vi "1,3A PWM-MotorControl and VBattSense FPGA.vi"() -> ()   [LabVIEW 2011]
doc: "FPGA VI for motor control and VBAttery Sensing.\n\nMotor Control:\nBoth servos are linked to seperate I/O terminals. The Generate Digital Pulse VI inouts the PUlsewidth in us (outputted by the 1.3A PWM Motor Control VI) and creates corresponding pulses on the pins. The clock timer determines the PWM cycle time."
uses:
  TestCode/spiTest/FPGA/Controls/Port Action.ctl
  <vilib>/Platform/TimedLoop/XDataNode/timing_clust.ctl
  <vilib>/Platform/TimedLoop/XDataNode/nitl_modes.ctl
  <vilib>/Platform/TimedLoop/XDataNode/wakeup.ctl
  <vilib>/robotics/Utilities/FPGA Utilities/Generate Digital Pulse (uSec).vi
  <vilib>/rvi/eio/common/nirviEmuTemplateMethod_errors.vi
  <vilib>/Platform/TimedLoop/XDataNode/XDataNode.xnode
  <vilib>/eio/EIONode/EIONode.xnode
  <vilib>/robotics/Utilities/FPGA Utilities/NI_Robotics_FPGA Utilities.lvlib
  <vilib>/Platform/TimedLoop/XDataNode/XDNodeRunTimeDep.lvlib
panel:
  out "VBatt Sense Iterations":i32
  out "Averaged bitstring":bool[](array[boolean])
  in  "VBatt samples to average":u16=30
  out "vBatt ADC bits":u16
  in  "stop VBatt Sense":bool
  in  "SERVO 2 Duty (uSec)":u32
  in  "stop PWM":bool
  in  "SERVO 1 Duty (uSec)":u32
  # "IF YOU HAVE TROUBLE RUNNING THIS: \ncheck if you're running it on FPGA target"
  # "Winch"
  # "Rudder"
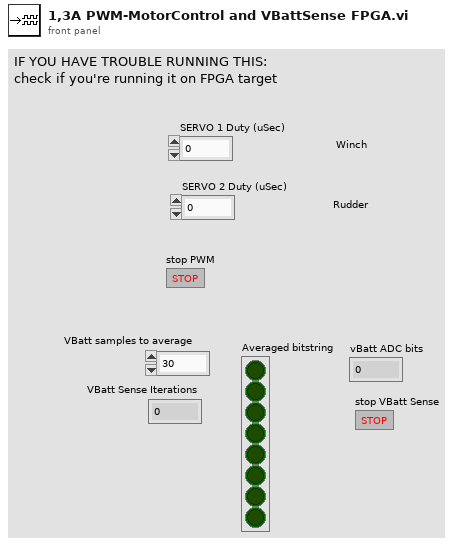
[diagram p1: front panel]
types:
  T1 = typedef "Port Action.ctl" = enum8{"Start Read", "Transition", "Wait Cycles", "End Read"}
  T2 = typedef "XDNodeRunTimeDep.lvlib/timing_clust.ctl" = cluster{"Expected End [f-1]":u64, "Actual End [f-1]":u64, "Finished Late? [f-1]":bool, "Expected End [i-1]":u64, "Actual End [i-1]":u64, "Finished Late? [i-1]":bool, "Expected Start [i]":u64, "Actual Start [i]":u64, "Expected Start [f]":u64, "Actual Start [f]":u64, "Source Name":string, "Structure Name":string, "Period":i64, "Deadline":i64, "Offset":i64, "Start":i64, "Priority":i32, "Timeout":i32, "Mode":T3, "Wakeup Reason":T4, "Error":errorcluster, "Source Type":string, "Secondary Source Type":string, "Global End Time":u64, "Global Start Time":u64, "Frame Duration":u64, "Iteration Duration":u64, "Assigned CPU":i32, "I/O Scan Engine Mode":u32}
  T3 = typedef "XDNodeRunTimeDep.lvlib/nitl_modes.ctl" = enum32{"No Change", "Process missed periods, maintain original phase", "Discard missed periods, maintain original phase", "Process missed periods, ignore original phase", "Discard missed periods, ignore original phase"}
  T4 = typedef "XDNodeRunTimeDep.lvlib/wakeup.ctl" = enum32{"Normal", "Aborted", "Asynchronous wakeup", "Timing source error", "Timed loop error", "Timeout"}
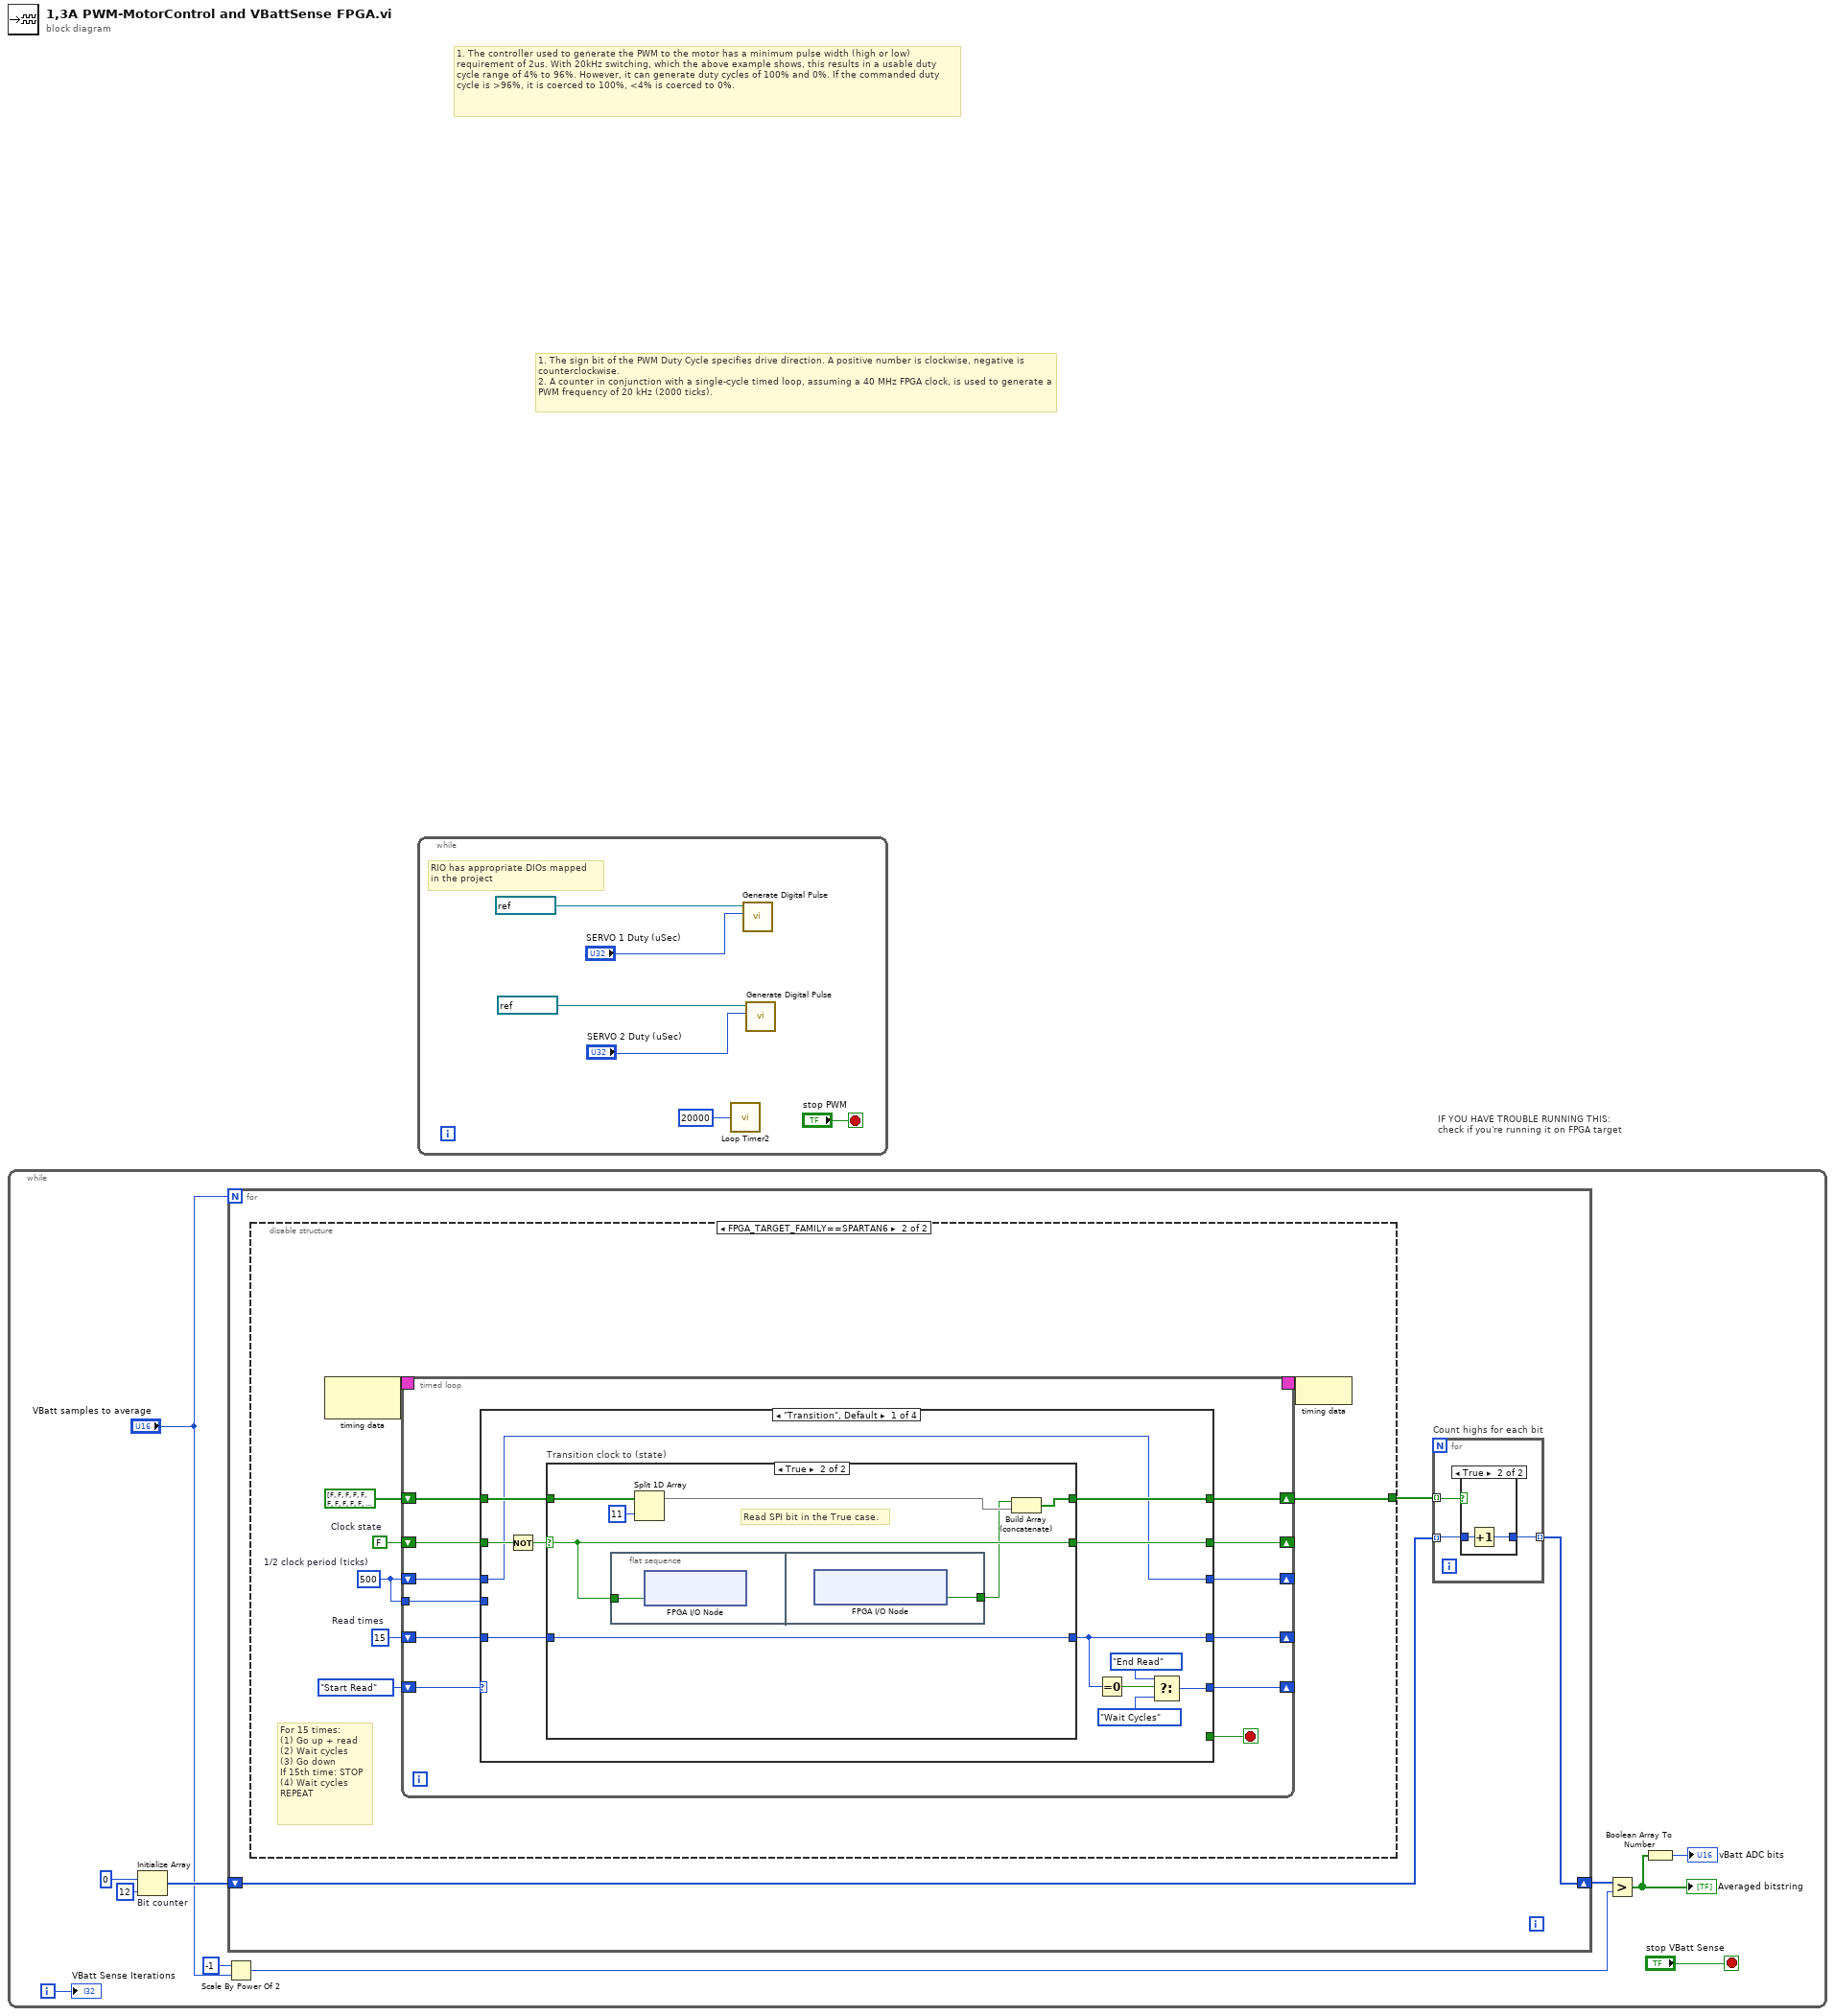
[diagram p0: block diagram]
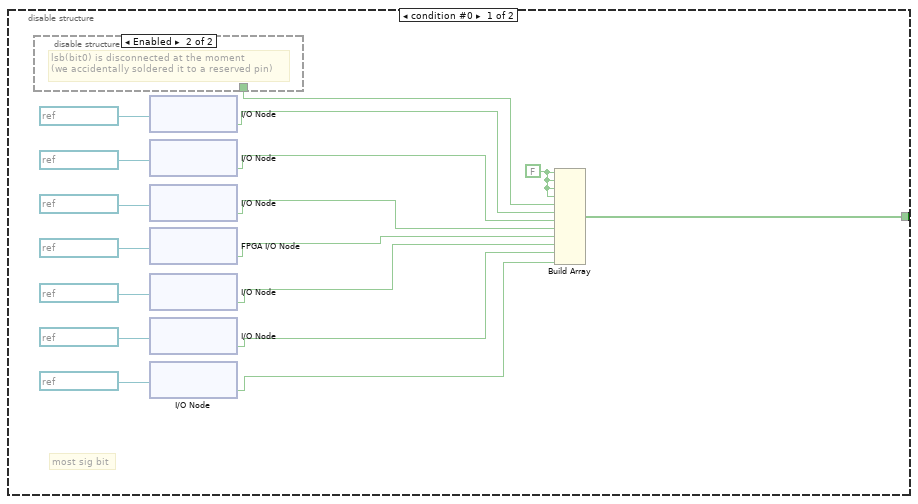
[diagram p2: hidden frame]
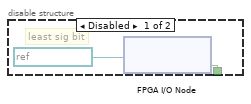
[diagram p3: hidden frame]
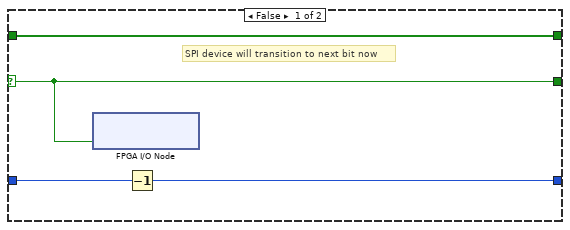
[diagram p4: hidden frame]
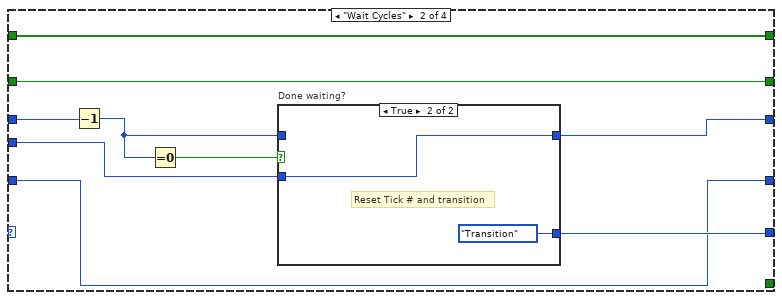
[diagram p5: hidden frame]
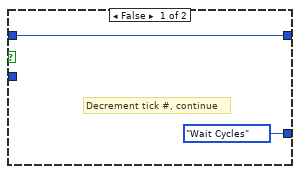
[diagram p6: hidden frame]
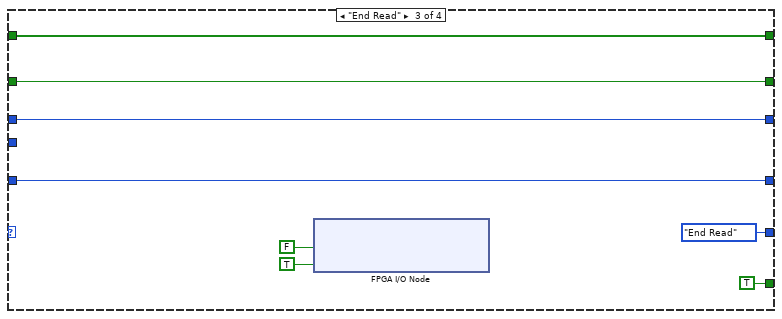
[diagram p7: hidden frame]
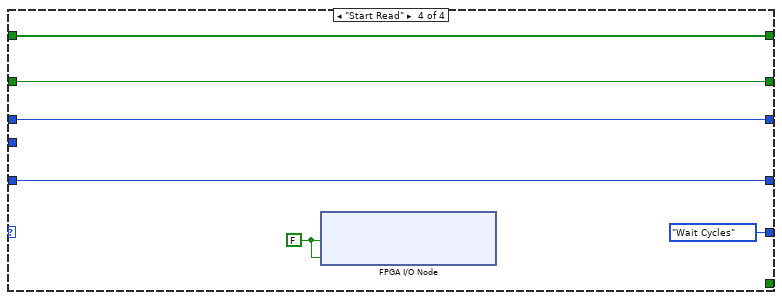
[diagram p8: hidden frame]
diagram:
  # "IF YOU HAVE TROUBLE RUNNING THIS: \ncheck if you're running it on FPGA target"
  # "1. The sign bit of the PWM Duty Cycle specifies drive direction. A positive number is clockwise, negative is counterclockwise.\n2. A counter in conjunction with a single-cycle timed loop, assuming a 40 MHz FPGA clock, is used to generate a PWM frequency of 20 kHz (2000 ticks)."
  # "1. The controller used to generate the PWM to the motor has a minimum pulse width (high or low) requirement of 2us. With 20kHz switching, which the above example shows, this results in a usable duty cycle range of 4% to 96%. However, it can generate duty cycles of 100% and 0%. If the commanded duty cycle is >96%, it is coerced to 100%, <4% is coerced to 0%."
  n1 = while {
    i -> [w8]
    stop <- "stop VBatt Sense" stop-if-true
    n2 = Initialize Array "Bit counter"(u16 0 ("VBatt Samples to read/2 2"), 12 ("dimension size")) -> (w5:u16[])
    n3 = Scale By Power Of 2(n=-1, x="VBatt samples to average") -> (x*2^n=w4:u16)
    n4 = for {
      N: "VBatt samples to average" -> [_]
      shift-right: [w12] -> w11
      shift-left: w5 -> [w14]
      n5 = disable-structure shown="FPGA_TARGET_FAMILY==SPARTAN6" {
        disable-tunnel: [w16 w34] -> w13
        frame condition #0 {
          w15 = FALSE ("element")
          # "most sig bit"
          n6 = disable-structure shown="Enabled" {
            disable-tunnel: [w32 _] -> w17
            frame Disabled {
              # "least sig bit"
              n7 = xnode "FPGA I/O Node"("FPGA I/O In"=refnum<k21> "VBatt bit0") -> ("I/O Item"=w32:bool)  [unwired: 1 out]
            }
            frame Enabled {
              # "lsb(bit0) is disconnected at the moment\n(we accidentally soldered it to a reserved pin)"
            }
          }
          n8 = xnode "I/O Node"("FPGA I/O In"=refnum<k21> "VBatt bit1") -> ("I/O Item"=w25:bool)  [unwired: 1 out]
          n9 = xnode "I/O Node"("FPGA I/O In"=refnum<k21> "VBatt bit2") -> ("I/O Item"=w26:bool)  [unwired: 1 out]
          n10 = xnode "I/O Node"("FPGA I/O In"=refnum<k21> "VBatt bit3") -> ("I/O Item"=w27:bool)  [unwired: 1 out]
          n11 = xnode "FPGA I/O Node"("FPGA I/O In"=refnum<k21> "VBatt bit4") -> ("I/O Item"=w28:bool)  [unwired: 1 out]
          n12 = xnode "I/O Node"("FPGA I/O In"=refnum<k21> "VBatt bit5") -> ("I/O Item"=w29:bool)  [unwired: 1 out]
          n13 = xnode "I/O Node"("FPGA I/O In"=refnum<k21> "VBatt bit6") -> ("I/O Item"=w30:bool)  [unwired: 1 out]
          n14 = xnode "I/O Node"("FPGA I/O In"=refnum<k21> "VBatt bit7") -> ("I/O Item"=w31:bool)  [unwired: 1 out]
          n15 = Build Array(w15, w15, w15, w15, w17, w25, w26, w27, w28, w29, w30, w31) -> (w16:bool[])
        }
        frame condition #1 (active) {
          w35 = u32 500  # 1/2 clock period (ticks)
          w36 = FALSE  # Clock state
          w37 = u8 15  # Read times
          # "For 15 times:\n(1) Go up + read\n(2) Wait cycles\n(3) Go down\nIf 15th time: STOP\n(4) Wait cycles\nREPEAT"
          n16 = node-c288() -> (w41:T2)  [unwired: 1 out]
          n17 = timed-loop {
            timing-out: [_] -> w40
            timing: w41 -> [_]
            shift-right: [w46] -> _
            shift-left: Port_Action."Start Read" ("Action") -> [w53]
            shift-right: [w49] -> w34
            shift-left: bool[] [FALSE, FALSE, FALSE, FALSE, FALSE, FALSE, FALSE, FALSE, FALSE, FALSE, FALSE, FALSE] ("Battery Voltage") -> [w50]
            shift-right: [w51] -> _
            shift-left: w36 -> [w52]
            tunnel: w35 -> [w44]
            shift-right: [w43] -> _
            shift-left: w35 -> [w45]
            shift-right: [w47] -> _
            shift-left: w37 -> [w48]
            stop <- w42 stop-if-true
            n18 = case shown="\"Transition\", Default" w53 {
              tunnel: w52 -> [w65 w87 w95 w103]
              tunnel: [w64 w87 w95 w103] -> w51
              tunnel: w50 -> [w62 w86 w94 w104]
              tunnel: [w61 w86 w94 w104] -> w49
              tunnel: w48 -> [w60 w79 w98 w101]
              tunnel: [w58 w79 w98 w101] -> w47
              tunnel: [w56 w82 Port_Action."End Read" ("Action") Port_Action."Wait Cycles" ("Action")] -> w46
              tunnel: w45 -> [w59 w85 w96 w102]
              tunnel: w44 -> [_ w80 _ _]
              tunnel: [w59 w81 w96 w102] -> w43
              tunnel: [_ _ TRUE _] -> w42
              frame "Transition", Default {
                n19 = Not(x=w65) -> (.not. x?=w63:bool)
                n20 = case "Transition clock to (state)" shown="True" w63 {
                  selector: w63 -> [w69 w76]
                  tunnel: [w69 w76] -> w64
                  tunnel: w62 -> [w66 w75]
                  tunnel: [w66 w73] -> w61
                  tunnel: w60 -> [w68 w72]
                  tunnel: [w67 w72] -> w58
                  frame False {
                    # "SPI device will transition to next bit now"
                    n21 = xnode "FPGA I/O Node"("VBatt_Clock"=w69) -> ()  [unwired: 1 in, 1 out]
                    n22 = Decrement(x=w68) -> (x-1=w67:u8)
                  }
                  frame True {
                    # "Read SPI bit in the True case."
                    n23 = flat-sequence {
                      tunnel: w76 -> [w77]
                      tunnel: [w78] -> w70
                      frame #0 {
                        n24 = xnode "FPGA I/O Node"("VBatt_Clock"=w77) -> ()  [unwired: 1 in, 1 out]
                      }
                      frame #1 {
                        n25 = xnode "FPGA I/O Node"() -> ("VBatt_DigitalInput"=w78:bool)  [unwired: 1 in, 1 out]
                      }
                    }
                    n26 = Split 1D Array(array=w75, index=11) -> (first subarray=w71:bool[])  [unwired: 1 out]
                    n27 = Build Array (concatenate)(w70, w71) -> (w73:bool[])
                  }
                }
                n28 = Equal To 0?(x=w58) -> (x = 0?=w57:bool)
                n29 = Select(t=Port_Action."End Read" ("Action"), s=w57, f=Port_Action."Wait Cycles" ("Action")) -> (s? t:f=w56:T1)
              }
              frame "Wait Cycles" {
                n30 = Decrement(x=w85) -> (x-1=w83:u32)
                n31 = Equal To 0?(x=w83) -> (x = 0?=w84:bool)
                n32 = case "Done waiting?" shown="True" w84 {
                  tunnel: w83 -> [w88 _]
                  tunnel: [Port_Action."Wait Cycles" ("Action") Port_Action."Transition" ("Action")] -> w82
                  tunnel: [w88 w90] -> w81
                  tunnel: w80 -> [_ w90]
                  frame False {
                    # "Decrement tick #, continue"
                  }
                  frame True {
                    # "Reset Tick # and transition"
                  }
                }
              }
              frame "End Read" {
                n33 = xnode "FPGA I/O Node"("VBatt_Clock"=FALSE ("VBatt_ChipSelectInverted"), "VBatt_ChipSelectInverted"=TRUE) -> ()  [unwired: 2 in, 2 out]
              }
              frame "Start Read" {
                w105 = FALSE ("VBatt_ChipSelectInverted")
                n34 = xnode "FPGA I/O Node"("VBatt_Clock"=w105, "VBatt_ChipSelectInverted"=w105) -> ()  [unwired: 2 in, 2 out]
              }
            }
          }
          n35 = node-c288(w40) -> ()
        }
      }
      n36 = for "Count highs for each bit" {
        tunnel: w13 -> [w112] mode=indexing
        tunnel: w14 -> [w111] mode=indexing
        tunnel: [w110] -> w12 mode=indexing
        n37 = case shown="True" w112 {
          tunnel: w111 -> [w113 w115]
          tunnel: [w113 w114] -> w110
          frame False {
          }
          frame True {
            n38 = Increment(x=w115) -> (x+1=w114:u16)
          }
        }
      }
    }
    n39 = Greater?(x=w11, y=w4) -> (0:w10:bool[])
    "Averaged bitstring" <- w10
    n40 = Boolean Array To Number(Boolean array=w10) -> (number=→"vBatt ADC bits":u16)
    "VBatt Sense Iterations" <- w8
  }
  n41 = while {
    stop <- "stop PWM" stop-if-true
    # "RIO has appropriate DIOs mapped\nin the project"
    n42 = call "Loop Timer2"("Count(uSec)"=u32 20000) -> ()  [unwired: 1 out]
    n43 = call-poly <vilib>:"Generate Digital Pulse.vi"("pulse width (uSec)"="SERVO 1 Duty (uSec)", "FPGA digital output"=refnum<k21> "Servo1") -> ()  [unwired: 10 in]
    n44 = call-poly <vilib>:"Generate Digital Pulse.vi"("pulse width (uSec)"="SERVO 2 Duty (uSec)", "FPGA digital output"=refnum<k21> "Servo2") -> ()  [unwired: 10 in]
  }
